vi "Format Nested Bullet List.vi"(8 "Error in":errorcluster caption="Error in (no error)", 10 "Delimiter (Tab)":string="\t", 11 "String Array":string[](array[string])) -> (0 "Error out":errorcluster, 3 "Nested Bullet List":string)   [LabVIEW 2023, in "Confluence Formatting.lvlib"]
uses:
  Confluence Formatting.lvlib
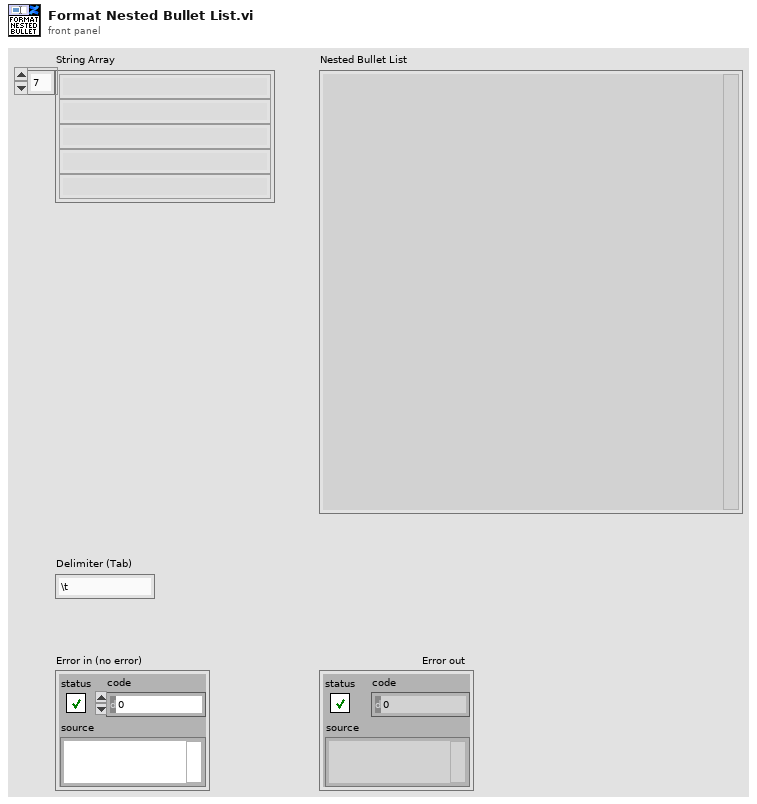
[diagram p1: front panel]
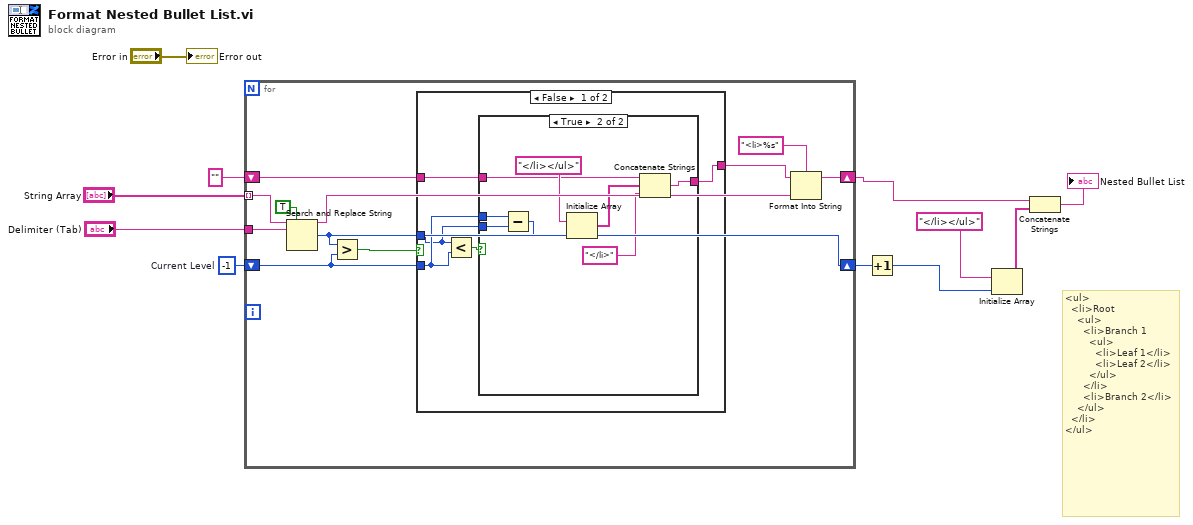
[diagram p0: block diagram]
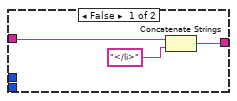
[diagram p2: hidden frame]
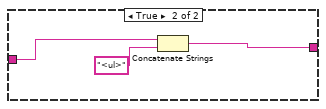
[diagram p3: hidden frame]
diagram:
  w7 = -1  # Current Level
  # "<ul>\n  <li>Root\n    <ul>\n      <li>Branch 1\n        <ul>\n          <li>Leaf 1</li>\n          <li>Leaf 2</li>\n        </ul>\n      </li>\n      <li>Branch 2</li>\n    </ul>\n  </li>\n</ul>"
  n1 = for {
    shift-right: [w22] -> w4
    shift-left: "" -> [w15]
    tunnel: "String Array" -> [w18] mode=indexing
    tunnel: "Delimiter (Tab)" -> [w20]
    shift-right: [w12] -> w5
    shift-left: w7 -> [w17]
    n2 = Search and Replace String(replace all?=TRUE ("replace all? (F)"), input string=w18, search string=w20) -> (result string=w19:string, number of replacements=w12:i32)  [unwired: 5 in, 2 out]
    n3 = Greater?(x=w12, y=w17) -> (0:w16:bool)
    n4 = case shown="False" w16 {
      tunnel: w12 -> [w24 _]
      tunnel: w17 -> [w25 _]
      tunnel: w15 -> [w26 w40]
      tunnel: [w23 w39] -> w14
      frame False {
        n5 = Less?(x=w24, y=w25) -> (x < y?=w27:bool)
        n6 = case shown="True" w27 {
          tunnel: w26 -> [w30 w34]
          tunnel: w25 -> [_ w38]
          tunnel: w24 -> [_ w37]
          tunnel: [w28 w32] -> w23
          frame False {
            n7 = Concatenate Strings(w30, "</li>" ("format string")) -> (w28:string)
          }
          frame True {
            n8 = Subtract(x=w38, y=w37) -> (x-y=w36:i32)
            n9 = Initialize Array("</li></ul>", w36) -> (w33:string[])
            n10 = Concatenate Strings(w34, w33, "</li>") -> (w32:string)
          }
        }
      }
      frame True {
        n11 = Concatenate Strings(w40, "<ul>") -> (w39:string)
      }
    }
    n12 = Format Into String(format string="<li>%s", initial string=w14, w19) -> (resulting string=w22:string)  [unwired: 1 in, 1 out]
  }
  n13 = Increment(x=w5) -> (x+1=w1:i32)
  n14 = Initialize Array("</li></ul>", w1) -> (w3:string[])
  n15 = Concatenate Strings(w4, w3) -> (→"Nested Bullet List":string)
  "Error out" <- "Error in"
